vi "autoconfigure mesh sync.vi"(1 "enable_mag":bool, 4 "enable_gyro":bool, 5 "enable_accel":bool, 6 "accel_full_scale_mode":bool, 7 "erase_sd_card":bool, 9 "enable_sd_card":bool, 10 "wireless_channel_number":u8, 11 "context":u32) -> (2 "function return":i32, 3 "context out":u32)   [LabVIEW 2019, in "apdm.lvlib"]
doc: "APDM_EXPORT int apdm_autoconfigure_mesh_sync(apdm_ctx_t context, const uint8_t wireless_channel_number,\n const bool enable_sd_card, const bool erase_sd_card,\n const bool accel_full_scale_mode, const bool enable_accel, const bool enable_gyro, const bool enable_mag);"
uses:
  apdm.lvlib
  Lee Lab/CP FES Walking 2018/Code/Working/LabVIEW/apdm.dll
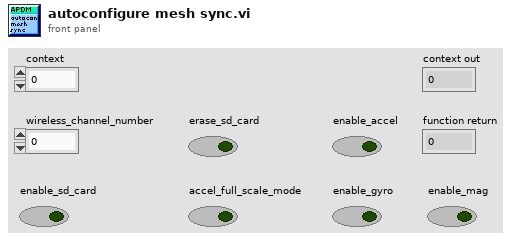
[diagram p1: front panel]
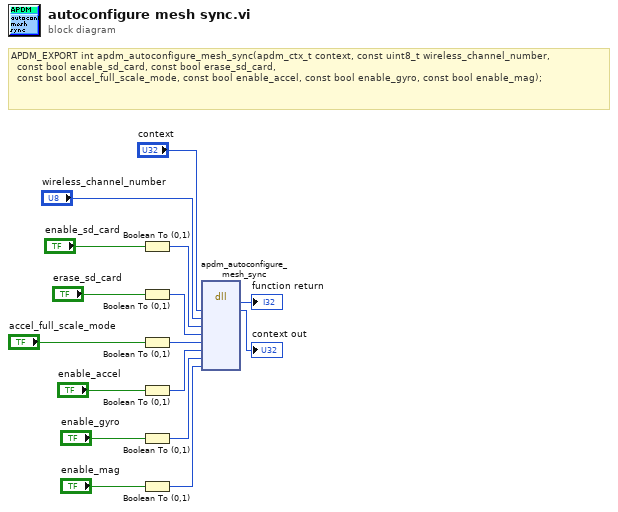
[diagram p0: block diagram]
diagram:
  # "APDM_EXPORT int apdm_autoconfigure_mesh_sync(apdm_ctx_t context, const uint8_t wireless_channel_number,\n\t\tconst bool enable_sd_card, const bool erase_sd_card,\n\t\tconst bool accel_full_scale_mode, const bool enable_accel, const bool enable_gyro, const bool enable_mag);"
  n1 = Boolean To (0,1)(Boolean="enable_sd_card") -> (0, 1=w11:i16)
  n2 = Boolean To (0,1)(Boolean="erase_sd_card") -> (0, 1=w9:i16)
  n3 = Boolean To (0,1)(Boolean="accel_full_scale_mode") -> (0, 1=w7:i16)
  n4 = Boolean To (0,1)(Boolean="enable_accel") -> (0, 1=w5:i16)
  n5 = Boolean To (0,1)(Boolean="enable_gyro") -> (0, 1=w3:i16)
  n6 = Boolean To (0,1)(Boolean="enable_mag") -> (0, 1=w1:i16)
  n7 = dll-call lib="C:/Users/jfalesi/Dropbox/Lee Lab/CP FES Walking 2018/Code/Working/LabVIEW/apdm.*" fn="apdm_autoconfigure_mesh_sync"("context"="context", "wireless_channel_number"="wireless_channel_number", "enable_sd_card"=w11, "erase_sd_card"=w9, "accel_full_scale_mode"=w7, "enable_accel"=w5, "enable_gyro"=w3, "enable_mag"=w1) -> (→"function return":i32, "context"=→"context out":u32)  [unwired: 10 in, 2 out]
